vi "setConfig.vi"(8 "error in (no error)":errorcluster, 11 "New Config":T1) -> (0 "error out":errorcluster)   [LabVIEW 2015, in "TPVG_DLL.lvlib"]
doc: "------------------------------------------\nAuthor: Dang Lam\nEmail: danglamtd@gmail.com"
uses:
  TPVG_DLL.lvlib
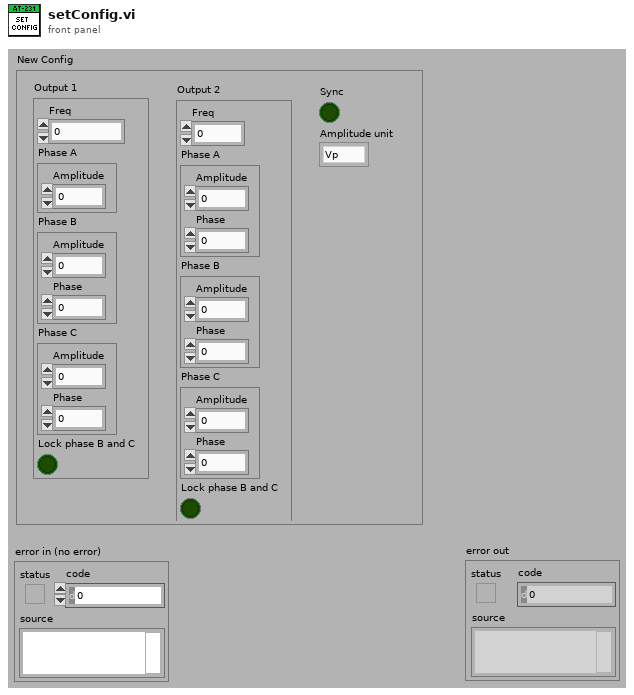
[diagram p1: front panel]
types:
  T1 = cluster{"Output 1":cluster{"Freq":sgl, "Phase A":cluster{"Amplitude":sgl}, "Phase B":cluster{"Amplitude":sgl, "Phase":sgl}, "Phase C":cluster{"Amplitude":sgl, "Phase":sgl}, "Lock":bool}, "Output 2":cluster{"Freq":sgl, "Phase A":cluster{"Amplitude":sgl, "Phase":sgl}, "Phase B":cluster{"Amplitude":sgl, "Phase":sgl}, "Phase C":cluster{"Amplitude":sgl, "Phase":sgl}, "Lock":bool}, "Sync":bool, "Amplitude unit":enum16{"Vp", "Vp-p", "Vrms"}}
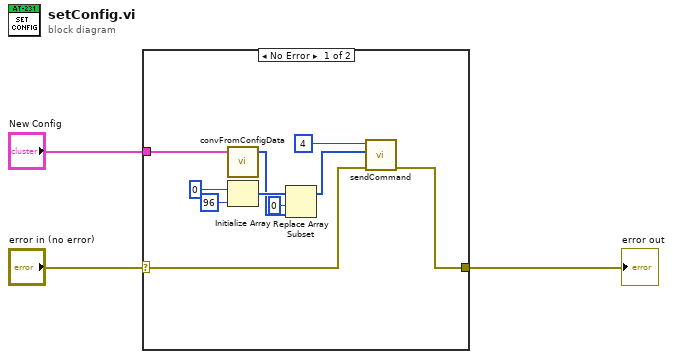
[diagram p0: block diagram]
diagram:
  n1 = case shown="No Error" "error in (no error)" {
    selector: "error in (no error)" -> [w12 w14]
    tunnel: [w11 w14] -> w2
    tunnel: "New Config" -> [w13 _]
    frame No Error {
      n2 = call "convFromConfigData.vi"("Config in"=w13) -> ("Config out"=w6:u8[])  [unwired: 4 in]
      n3 = Initialize Array(u8 0, 96 ("dimension size")) -> (w7:u8[])
      n4 = Replace Array Subset(array=w7, new element=w6, index=0) -> (w5:u8[])
      n5 = call "sendCommand.vi"("error in (no error)"=w12, "Data in"=w5, "Command ID"=u16 4) -> ("error out"=w11:errorcluster)  [unwired: 7 in, 1 out]
    }
    frame Error {
    }
  }
  "error out" <- w2
